vi "Enqueue.vi"(7 "Priority (f)":bool, 8 "ErrorArray In":errorcluster[](array[cluster]), 9 "Data":variant, 10 "Msg":string) -> (0 "ErrorArray Out":errorcluster[](array[cluster]))   [LabVIEW 2014, in "TestFramework.lvlib"]
uses:
  TestFramework.lvlib
  TypeDef/MsgQueue.ctl
  <userlib>/NIST/NISTErrorLib/NISTErrorLib.lvlib
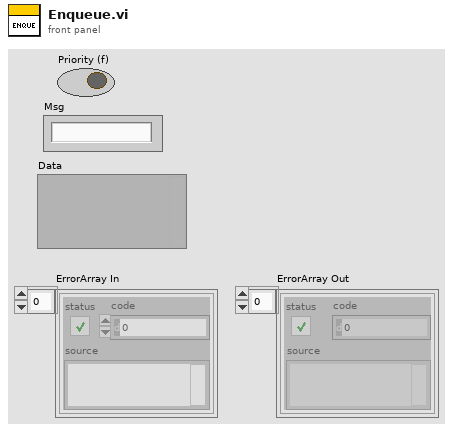
[diagram p1: front panel]
types:
  T1 = typedef "TestFramework.lvlib/MsgQueue.ctl" = cluster{"Msg":string, "Data":variant}
  T2 = typedef "TestFramework.lvlib/QueRef.ctl" = refnum<queue>
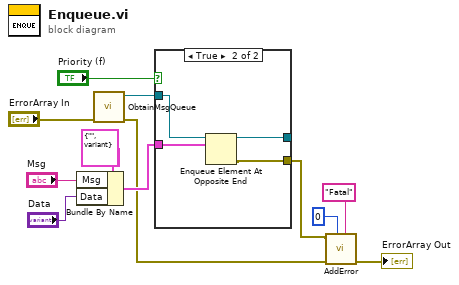
[diagram p0: block diagram]
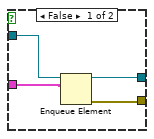
[diagram p2: hidden frame]
diagram:
  n1 = Bundle By Name(cluster=T1 {"Msg"="", "Data"=variant} ("MsgQueue"), "Msg"="Msg", "Data"="Data") -> (w5:T1)
  n2 = call "ObtainMsgQueue.vi"("ErrorArray In"="ErrorArray In") -> ("ErrorArray Out"=w1:errorcluster[], "QueRef"=w2:T2)  [unwired: 9 in]
  n3 = case shown="True" "Priority (f)" {
    tunnel: w5 -> [w16 w20]
    tunnel: [w15 w19] -> w4
    tunnel: w2 -> [w14 w18]
    tunnel: [w13 w17] -> _
    frame False {
      n4 = Enqueue Element(queue=w14, element=w16) -> (queue out=w13:T2, error out=w15:errorcluster)  [unwired: 2 in, 1 out]
    }
    frame True {
      n5 = Enqueue Element At Opposite End(queue=w18, element=w20) -> (queue out=w17:T2, error out=w19:errorcluster)  [unwired: 2 in, 1 out]
    }
  }
  n6 = call <userlib>:"AddError.vi"("Severity"="Fatal", "Priority"=u8 0, "ErrorArray"=w1, "error in (no error)"=w4) -> ("ErrorArray"=→"ErrorArray Out":errorcluster[])  [unwired: 6 in, 1 out]
